vi "Delete Initialize VIs.vi"   [LabVIEW 2015]
uses:
  Project Manipulation Scripts/Project Manipulation Scripts.lvlib
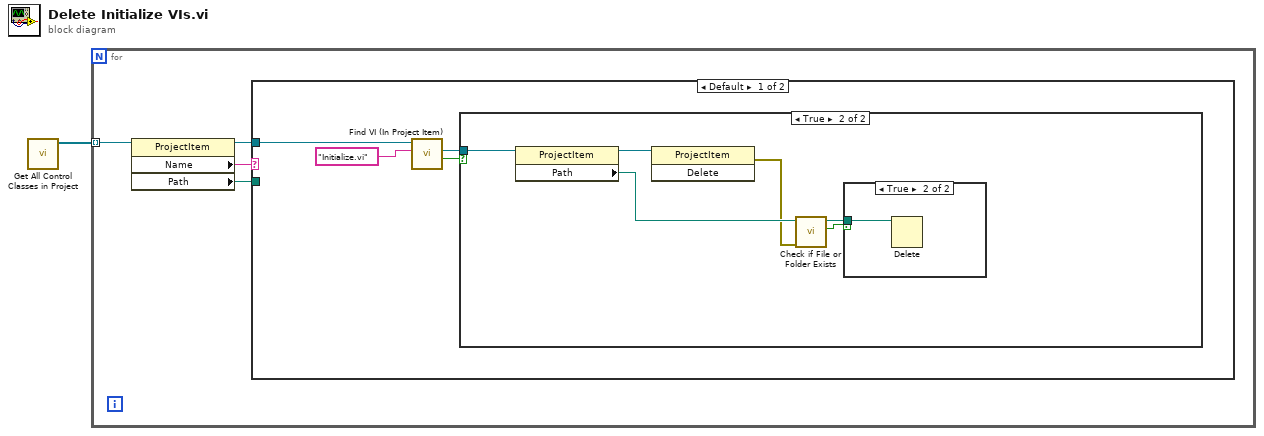
[diagram p0: block diagram]
diagram:
  n1 = call "Get All Control Classes in Project.vi"() -> ("All Control Classes"=w1:refnum<vi>[])  [unwired: 11 in]
  n2 = for {
    tunnel: w1 -> [w5] mode=indexing
    n3 = property class="ProjectItem"(reference=w5) -> (reference out=w3:refnum<vi>, "Name"=w4:string, "Path"=w2:path)  [unwired: 1 in, 1 out]
    n4 = case shown="Default" w4 {
      tunnel: w3 -> [w9 _]
      tunnel: w2 -> [_ _]
      frame Default {
        n5 = call "Find VI (In Project Item).vi"("VI Name"="Initialize.vi" ("format string"), "ProjectItem in"=w9) -> ("Found?"=w7:bool, "VI ProjectItem Refnum"=w8:refnum<vi>)  [unwired: 7 in, 1 out]
        n6 = case shown="True" w7 {
          tunnel: w8 -> [_ w12]
          frame False {
          }
          frame True {
            n7 = property class="ProjectItem"(reference=w12) -> (reference out=w11:refnum<vi>, "Path"=w15:path)  [unwired: 1 in, 1 out]
            n8 = invoke class="ProjectItem" method="Delete"(reference=w11) -> (error out=w10:errorcluster)  [unwired: 2 in, 2 out]
            n9 = call <vilib>:"Check if File or Folder Exists.vi"("error in (no error)"=w10, "path"=w15) -> ("file or folder exists?"=w13:bool, "dup path"=w14:path)  [unwired: 7 in, 1 out]
            n10 = case shown="True" w13 {
              tunnel: w14 -> [_ w16]
              frame False {
              }
              frame True {
                n11 = Delete(path (use dialog)=w16) -> ()  [unwired: 4 in, 3 out]
              }
            }
          }
        }
      }
      frame "Control.lvclass" {
      }
    }
  }
